vi "CMN_CalcDetReadTime.vi"(0 "Det Columns":i32, 1 "Pixel Read Time (usecs)":dbl format="%.3f", 2 "Serial Skip Time (usecs)":dbl format="%.3f", 3 "skips_per_row_shift":i32, 4 "y roi start":i32, 5 "Det Rows":i32, 7 "cols":i32, 9 "rows":i32, 10 "num of X amps":u16=1, 11 "Num of amps":u32=1, 12 "Paralel Shift Time (usecs)":dbl format="%.3f", 13 "Parallel Skip Time (usecs)":dbl format="%.3f", 14 "overhead":sgl format="%.3f", 15 "num of Y amps":u16=1) -> (8 "Timing_out":T1 {"Total Read Time" format="%.3f"; "Total Paralel shift time" format="%.3f"; "Total Paralel skip time" format="%.3f"; "Total serial skip time" format="%.3f"; "Total Pixel read time" format="%.3f"})   [LabVIEW 2016]
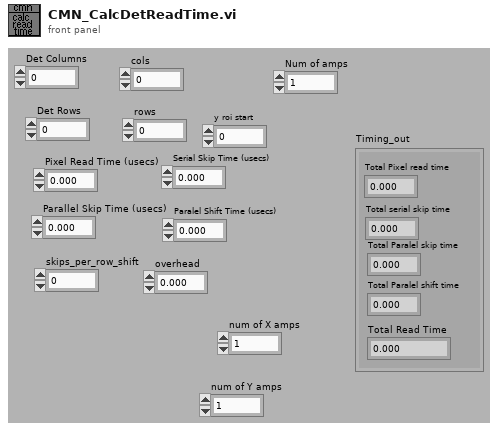
[diagram p1: front panel]
types:
  T1 = cluster{"Total Pixel read time":dbl, "Total serial skip time":dbl, "Total Paralel skip time":dbl, "Total Paralel shift time":dbl, "Total Read Time":dbl}
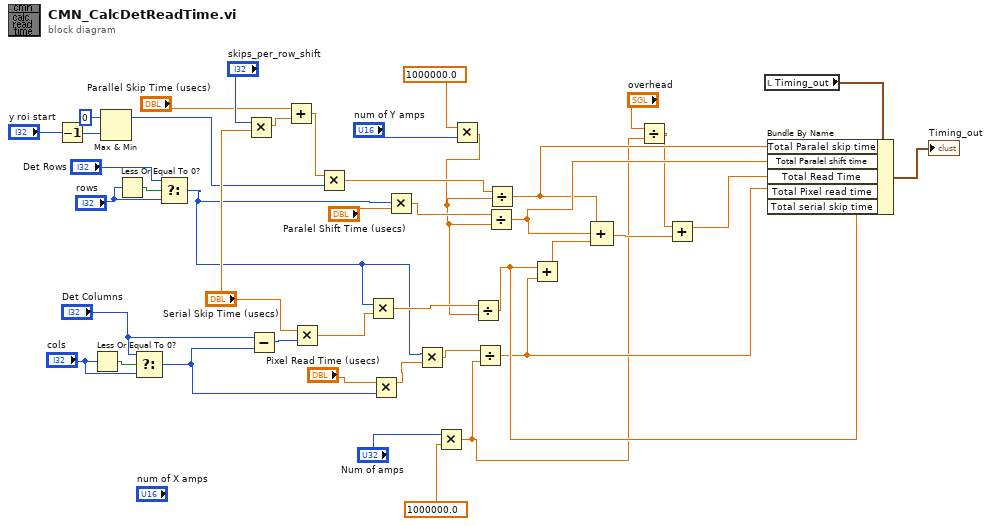
[diagram p0: block diagram]
diagram:
  n1 = Decrement(x="y roi start") -> (x-1=w9:i32)
  n2 = Less Or Equal To 0?(x="cols") -> (x <= 0?=w39:bool)
  n3 = Max & Min(x=0, y=w9) -> (max(x,y)=w6:i32)  [unwired: 1 out]
  n4 = Less Or Equal To 0?(x="rows") -> (x <= 0?=w36:bool)
  n5 = Select(t="Det Columns", s=w39, f="cols") -> (s? t:f=w37:i32)
  n6 = Select(t="Det Rows", s=w36, f="rows") -> (s? t:f=w7:i32)
  n7 = Multiply(x="skips_per_row_shift", y="Serial Skip Time (usecs)") -> (x*y=w31:dbl)
  n8 = Subtract(x="Det Columns", y=w37) -> (x-y=w43:i32)
  n9 = Add(x="Parallel Skip Time (usecs)", y=w31) -> (x+y=w29:dbl)
  n10 = Multiply(x="Serial Skip Time (usecs)", y=w43) -> (x*y=w27:dbl)
  n11 = Multiply(x=w29, y=w6) -> (x*y=w26:dbl)
  n12 = Multiply(x=w7, y=w27) -> (x*y=w24:dbl)
  n13 = Multiply(x="Pixel Read Time (usecs)", y=w37) -> (x*y=w28:dbl)
  n14 = Multiply(x=w7, y="Paralel Shift Time (usecs)") -> (x*y=w25:dbl)
  n15 = Multiply(x=w7, y=w28) -> (x*y=w23:dbl)
  n16 = Multiply(x="Num of amps", y=1000000.0) -> (x*y=w1:dbl)
  n17 = Multiply(x=1000000.0 ("y"), y="num of Y amps") -> (x*y=w2:dbl)
  n18 = Divide(x=w24, y=w2) -> (x/y=w18:dbl)
  n19 = Divide(x=w23, y=w1) -> (x/y=w15:dbl)
  n20 = Divide(x=w25, y=w2) -> (x/y=w17:dbl)
  n21 = Divide(x=w26, y=w2) -> (x/y=w16:dbl)
  n22 = Add(x=w18, y=w15) -> (x+y=w22:dbl)
  n23 = Compound Arithmetic op=ADD(w16, w17, w22) -> (w21:dbl)
  n24 = Divide(x="overhead", y=w1) -> (x/y=w12:dbl)
  n25 = Add(x=w12, y=w21) -> (x+y=w14:dbl)
  n26 = local read "Timing_out"() -> (w19:T1)
  n27 = Bundle By Name(cluster=w19, "Total Paralel skip time"=w16, "Total Paralel shift time"=w17, "Total Read Time"=w14, "Total Pixel read time"=w15, "Total serial skip time"=w18) -> (→"Timing_out":T1)
